vi "InitCCLM.vi"(0 "COM Port Select":refnum<visa-resource-name>, 5 "StartModeEnable":bool=TRUE, 9 "error in (no error)":errorcluster, 11 "User control":T1={"Stimulation Parameters"={"Amplitude (mA)"={"A1"=1, "A2"=0, "A3"=0, "A4"=0, "A5"=0, "A6"=0, "A7"=0, "A8"=0}, "Pulse Width (µs)"={"PW1"=20, "PW2"=20, "PW3"=20, "PW4"=20, "PW5"=20, "PW6"=20, "PW7"=20, "PW8"=20}, "Stimulation Mode"={"M1"=0, "M2"=0, "M3"=0, "M4"=0, "M5"=0, "M6"=0, "M7"=0, "M8"=0}}, "Waveform Parameters"={"Low Frequency Factor"=0, "Main Stim Interval [ms]"=8.0, "Interpulse Interval [ms]"=0, "Channel Execution"=0}, "Active channels"={"C1"=FALSE, "C2"=FALSE, "C3"=FALSE, "C4"=FALSE, "C5"=FALSE, "C6"=FALSE, "C7"=FALSE, "C8"=FALSE}, "LF Active Channels"={"LF1"=FALSE, "LF2"=FALSE, "LF3"=FALSE, "LF4"=FALSE, "LF5"=FALSE, "LF6"=FALSE, "LF7"=FALSE, "LF8"=FALSE}, "Device Control"={"VISA resource name"=""}} {"Stimulation Parameters"."Amplitude (mA)"."A1" max=130; "Stimulation Parameters"."Amplitude (mA)"."A2" max=130; "Stimulation Parameters"."Amplitude (mA)"."A3" max=130; "Stimulation Parameters"."Amplitude (mA)"."A4" max=130; "Stimulation Parameters"."Amplitude (mA)"."A5" max=130; "Stimulation Parameters"."Amplitude (mA)"."A6" max=130; "Stimulation Parameters"."Amplitude (mA)"."A7" max=130; "Stimulation Parameters"."Amplitude (mA)"."A8" max=130; "Stimulation Parameters"."Pulse Width (µs)"."PW1" min=20 max=500; "Stimulation Parameters"."Pulse Width (µs)"."PW2" min=20 max=500; "Stimulation Parameters"."Pulse Width (µs)"."PW3" min=20 max=500; "Stimulation Parameters"."Pulse Width (µs)"."PW4" min=20 max=500; "Stimulation Parameters"."Pulse Width (µs)"."PW5" min=20 max=500; "Stimulation Parameters"."Pulse Width (µs)"."PW6" min=20 max=500; "Stimulation Parameters"."Pulse Width (µs)"."PW7" min=20 max=500; "Stimulation Parameters"."Pulse Width (µs)"."PW8" min=20 max=500; "Stimulation Parameters"."Stimulation Mode"."M8" items=["Singlet", "Doublet", "Triplet"]; "Stimulation Parameters"."Stimulation Mode"."M7" items=["Singlet", "Doublet", "Triplet"]; "Stimulation Parameters"."Stimulation Mode"."M6" items=["Singlet", "Doublet", "Triplet"]; "Stimulation Parameters"."Stimulation Mode"."M5" items=["Singlet", "Doublet", "Triplet"]; "Stimulation Parameters"."Stimulation Mode"."M4" items=["Singlet", "Doublet", "Triplet"]; "Stimulation Parameters"."Stimulation Mode"."M3" items=["Singlet", "Doublet", "Triplet"]; "Stimulation Parameters"."Stimulation Mode"."M2" items=["Singlet", "Doublet", "Triplet"]; "Stimulation Parameters"."Stimulation Mode"."M1" items=["Singlet", "Doublet", "Triplet"]; "Waveform Parameters"."Channel Execution" items=["Fixed Interval", "ASAP"]}) -> (3 "Status":string, 4 "VISA resource name out":refnum<visa-resource-name>, 6 "Stimulation Initialized":bool=TRUE, 14 "CCLM Initialization Error":bool=TRUE, 15 "error out":errorcluster)   [LabVIEW 2020]
uses:
  Type Defs/rs2_ctrl_panel.ctl
panel:
  out "Packet Number Out":i32
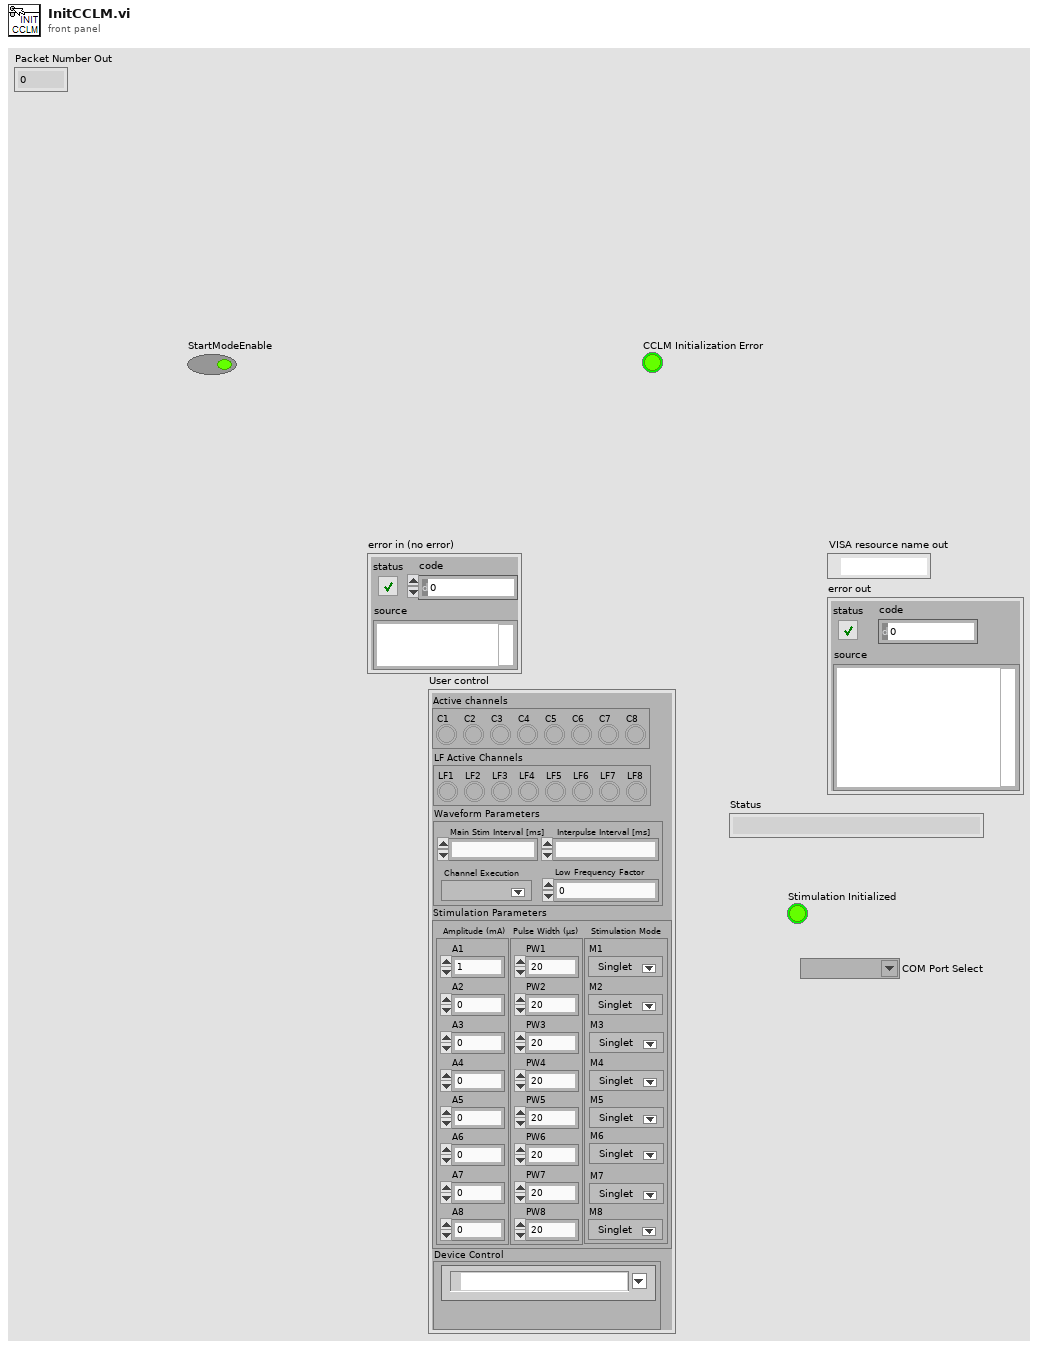
[diagram p1: front panel]
types:
  T1 = typedef "rs2_ctrl_panel.ctl" = cluster{"Stimulation Parameters":cluster{"Amplitude (mA)":cluster{"A1":u8, "A2":u8, "A3":u8, "A4":u8, "A5":u8, "A6":u8, "A7":u8, "A8":u8}, "Pulse Width (µs)":cluster{"PW1":u16, "PW2":u16, "PW3":u16, "PW4":u16, "PW5":u16, "PW6":u16, "PW7":u16, "PW8":u16}, "Stimulation Mode":cluster{"M1":u8, "M2":u8, "M3":u8, "M4":u8, "M5":u8, "M6":u8, "M7":u8, "M8":u8}}, "Waveform Parameters":cluster{"Low Frequency Factor":u8, "Main Stim Interval [ms]":fxp<+,32,11>, "Interpulse Interval [ms]":u8, "Channel Execution":u8}, "Active channels":cluster{"C1":bool, "C2":bool, "C3":bool, "C4":bool, "C5":bool, "C6":bool, "C7":bool, "C8":bool}, "LF Active Channels":cluster{"LF1":bool, "LF2":bool, "LF3":bool, "LF4":bool, "LF5":bool, "LF6":bool, "LF7":bool, "LF8":bool}, "Device Control":cluster{"VISA resource name":refnum<visa-resource-name>}}
  T2 = cluster{"Low Frequency Factor":u8, "Main Stim Interval [ms]":fxp<+,32,11>, "Interpulse Interval [ms]":u8, "Channel Execution":u8}
  T3 = cluster{"C1":bool, "C2":bool, "C3":bool, "C4":bool, "C5":bool, "C6":bool, "C7":bool, "C8":bool}
  T4 = cluster{"LF1":bool, "LF2":bool, "LF3":bool, "LF4":bool, "LF5":bool, "LF6":bool, "LF7":bool, "LF8":bool}
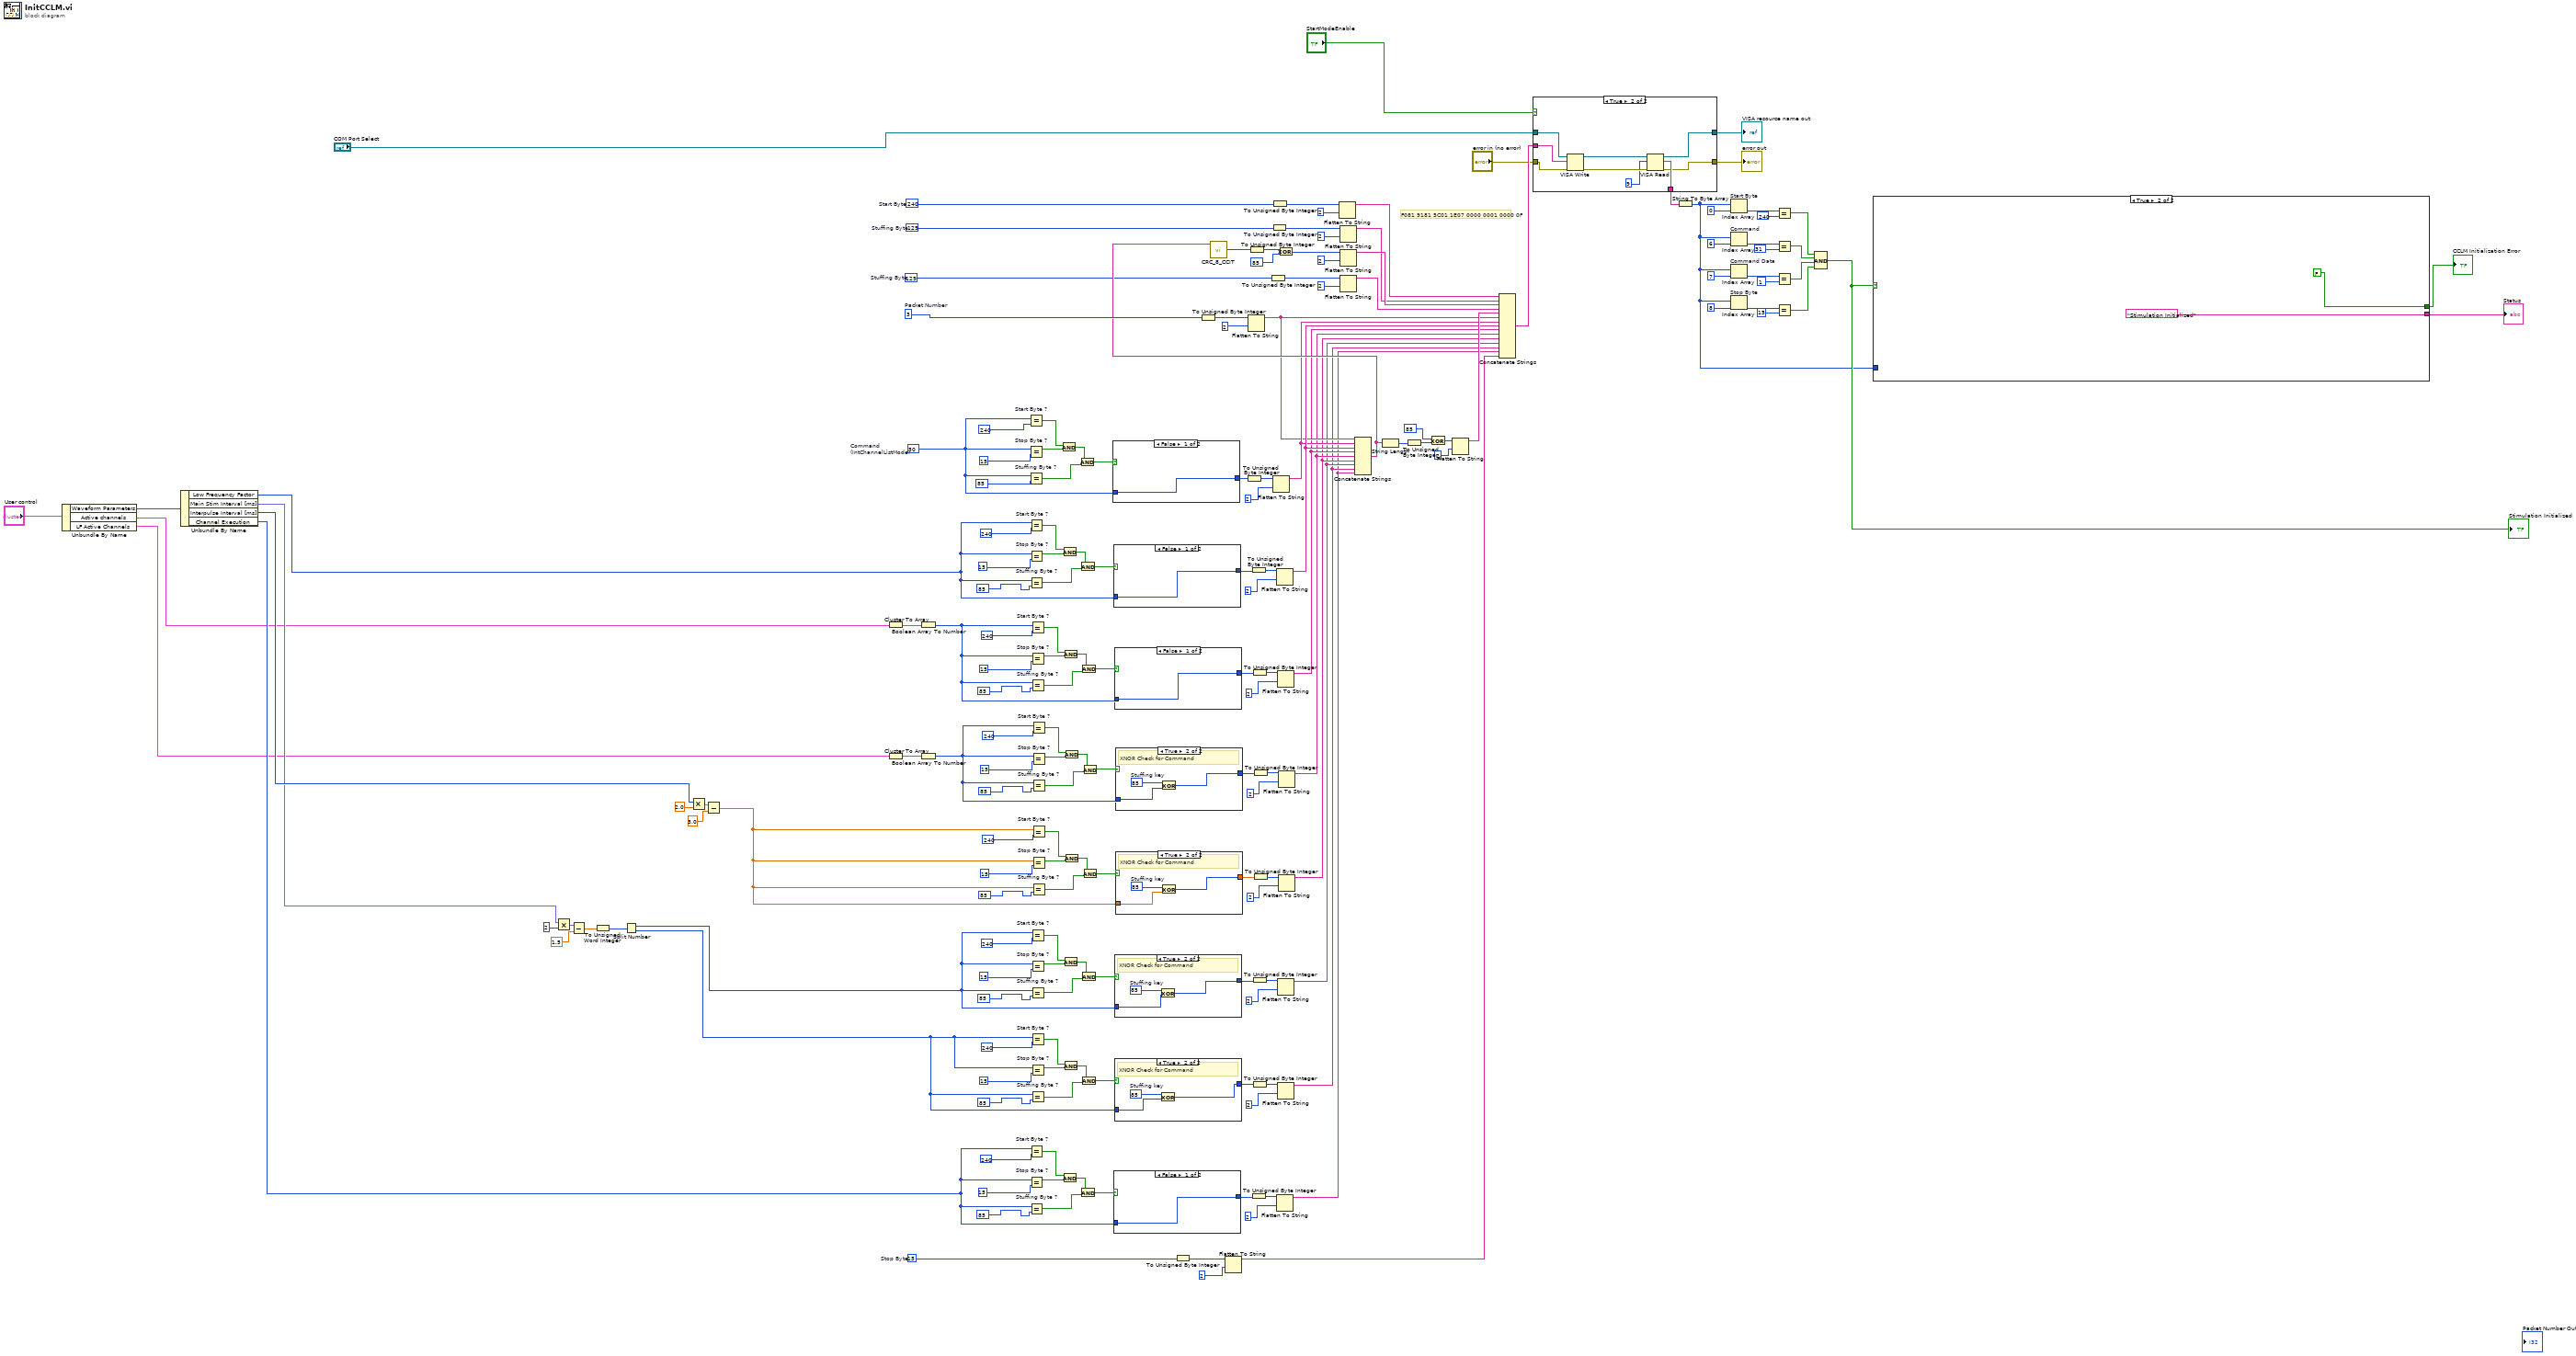
[diagram p0: block diagram]
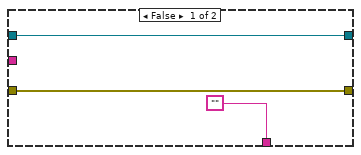
[diagram p2: hidden frame]
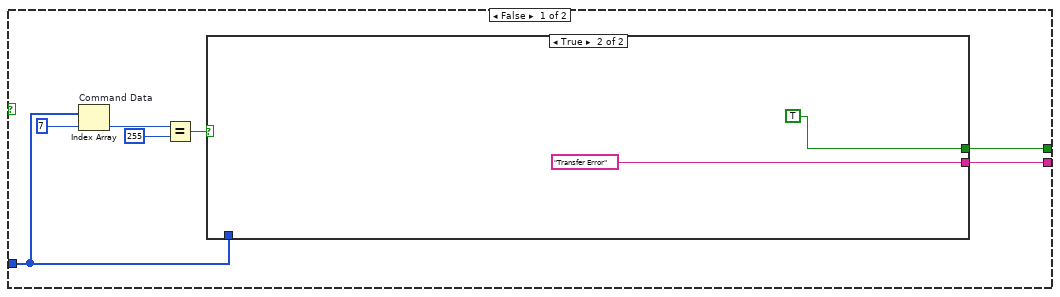
[diagram p3: hidden frame]
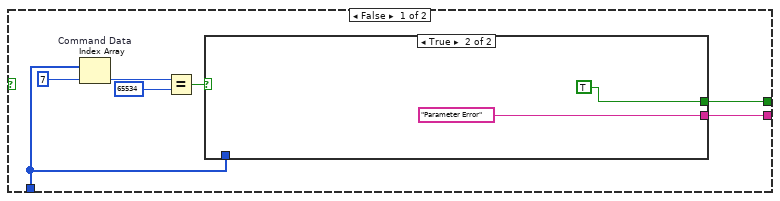
[diagram p4: hidden frame]
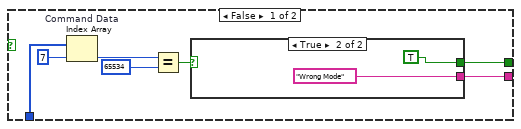
[diagram p5: hidden frame]
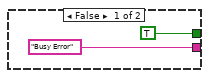
[diagram p6: hidden frame]
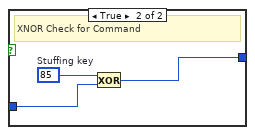
[diagram p7: hidden frame]
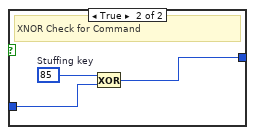
[diagram p12: hidden frame]
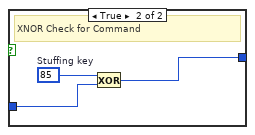
[diagram p13: hidden frame]
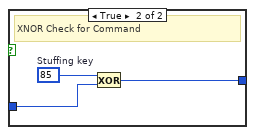
[diagram p14: hidden frame]
diagram:
  w178 = u8 3  # Packet Number
  w135 = 15  # Stop Byte
  w138 = 129  # Stuffing Byte
  w139 = 129  # Stuffing Byte
  w137 = 240  # Start Byte
  w157 = 30  # Command (IntChannelListMode)
  # "F081 9181 5C01 1E07 0000 0001 0000 0F"
  n1 = Unbundle By Name("User control") -> ("Waveform Parameters"=w10:T2, "Active channels"=w5:T3, "LF Active Channels"=w4:T4)
  n2 = Unbundle By Name(w10) -> ("Low Frequency Factor"=w9:u8, "Main Stim Interval [ms]"=w7:fxp<+,32,11>, "Interpulse Interval [ms]"=w8:u8, "Channel Execution"=w6:u8)
  n3 = Multiply(x=w7, y=u8 2) -> (x*y=w35:fxp<+,40,19>)
  n4 = Subtract(x=w35, y=1.5) -> (x-y=w32:dbl)
  n5 = To Unsigned Word Integer(number=w32) -> (unsigned 16bit integer=w33:u16)
  n6 = Split Number(x=w33) -> (hi(x)=w39:u8, lo(x)=w38:u8)
  n7 = Multiply(x=w8, y=2.0) -> (x*y=w42:dbl)
  n8 = Subtract(x=w42, y=3.0) -> (x-y=w40:dbl)
  n9 = Cluster To Array(cluster=w5) -> (array=w48:bool[])
  n10 = Cluster To Array(cluster=w4) -> (array=w44:bool[])
  n11 = Boolean Array To Number(Boolean array=w48) -> (number=w46:u8)
  n12 = Boolean Array To Number(Boolean array=w44) -> (number=w47:u8)
  n13 = Equal? "Start Byte ?"(x=w157, y=240 ("IntAck")) -> (x = y?=w121:bool)
  n14 = Equal? "Stop Byte ?"(x=w157, y=15 ("IntAck")) -> (x = y?=w122:bool)
  n15 = Equal? "Stuffing Byte ?"(x=w157, y=85 ("IntAck")) -> (x = y?=w124:bool)
  n16 = Equal? "Start Byte ?"(x=w9, y=240 ("IntAck")) -> (x = y?=w126:bool)
  n17 = Equal? "Stop Byte ?"(x=w9, y=15 ("IntAck")) -> (x = y?=w127:bool)
  n18 = Equal? "Stuffing Byte ?"(x=w9, y=85 ("IntAck")) -> (x = y?=w129:bool)
  n19 = Equal? "Start Byte ?"(x=w6, y=240 ("IntAck")) -> (x = y?=w56:bool)
  n20 = Equal? "Stop Byte ?"(x=w6, y=15 ("IntAck")) -> (x = y?=w57:bool)
  n21 = Equal? "Stuffing Byte ?"(x=w6, y=85 ("IntAck")) -> (x = y?=w59:bool)
  n22 = Equal? "Start Byte ?"(x=w46, y=240 ("IntAck")) -> (x = y?=w110:bool)
  n23 = Equal? "Stop Byte ?"(x=w46, y=15 ("IntAck")) -> (x = y?=w111:bool)
  n24 = Equal? "Stuffing Byte ?"(x=w46, y=85 ("IntAck")) -> (x = y?=w113:bool)
  n25 = Equal? "Start Byte ?"(x=w39, y=240 ("IntAck")) -> (x = y?=w77:bool)
  n26 = Equal? "Stop Byte ?"(x=w39, y=15 ("IntAck")) -> (x = y?=w78:bool)
  n27 = Equal? "Stuffing Byte ?"(x=w39, y=85 ("IntAck")) -> (x = y?=w80:bool)
  n28 = Equal? "Start Byte ?"(x=w38, y=240 ("IntAck")) -> (x = y?=w67:bool)
  n29 = Equal? "Stop Byte ?"(x=w38, y=15 ("IntAck")) -> (x = y?=w68:bool)
  n30 = Equal? "Stuffing Byte ?"(x=w38, y=85 ("IntAck")) -> (x = y?=w70:bool)
  n31 = Equal? "Start Byte ?"(x=w47, y=240 ("IntAck")) -> (x = y?=w99:bool)
  n32 = Equal? "Stop Byte ?"(x=w47, y=15 ("IntAck")) -> (x = y?=w100:bool)
  n33 = Equal? "Stuffing Byte ?"(x=w47, y=85 ("IntAck")) -> (x = y?=w102:bool)
  n34 = Equal? "Start Byte ?"(x=w40, y=240 ("IntAck")) -> (x = y?=w88:bool)
  n35 = Equal? "Stop Byte ?"(x=w40, y=15 ("IntAck")) -> (x = y?=w89:bool)
  n36 = Equal? "Stuffing Byte ?"(x=w40, y=85 ("IntAck")) -> (x = y?=w91:bool)
  n37 = And(x=w121, y=w122) -> (x .and. y?=w123:bool)
  n38 = And(x=w126, y=w127) -> (x .and. y?=w128:bool)
  n39 = And(x=w56, y=w57) -> (x .and. y?=w58:bool)
  n40 = And(x=w110, y=w111) -> (x .and. y?=w112:bool)
  n41 = And(x=w77, y=w78) -> (x .and. y?=w79:bool)
  n42 = And(x=w67, y=w68) -> (x .and. y?=w69:bool)
  n43 = And(x=w99, y=w100) -> (x .and. y?=w101:bool)
  n44 = And(x=w88, y=w89) -> (x .and. y?=w90:bool)
  n45 = And(x=w123, y=w124) -> (x .and. y?=w125:bool)
  n46 = And(x=w128, y=w129) -> (x .and. y?=w130:bool)
  n47 = And(x=w58, y=w59) -> (x .and. y?=w60:bool)
  n48 = And(x=w112, y=w113) -> (x .and. y?=w114:bool)
  n49 = And(x=w79, y=w80) -> (x .and. y?=w81:bool)
  n50 = And(x=w69, y=w70) -> (x .and. y?=w71:bool)
  n51 = And(x=w101, y=w102) -> (x .and. y?=w103:bool)
  n52 = And(x=w90, y=w91) -> (x .and. y?=w92:bool)
  n53 = case shown="False" w125 {
    tunnel: w157 -> [w181 w184]
    tunnel: [w181 w182] -> w159
    frame False {
    }
    frame True {
      w183 = 85  # Stuffing key
      # "XNOR Check for Command"
      n54 = Exclusive Or(1:w184, 2:w183) -> (0:w182:i32)
    }
  }
  n55 = case shown="False" w130 {
    tunnel: w9 -> [w185 w188]
    tunnel: [w185 w186] -> w158
    frame False {
    }
    frame True {
      w187 = 85  # Stuffing key
      # "XNOR Check for Command"
      n56 = Exclusive Or(1:w188, 2:w187) -> (0:w186:i32)
    }
  }
  n57 = case shown="False" w60 {
    tunnel: w6 -> [w189 w192]
    tunnel: [w189 w190] -> w65
    frame False {
    }
    frame True {
      w191 = 85  # Stuffing key
      # "XNOR Check for Command"
      n58 = Exclusive Or(1:w192, 2:w191) -> (0:w190:i32)
    }
  }
  n59 = case shown="False" w114 {
    tunnel: w46 -> [w193 w196]
    tunnel: [w193 w194] -> w119
    frame False {
    }
    frame True {
      w195 = 85  # Stuffing key
      # "XNOR Check for Command"
      n60 = Exclusive Or(1:w196, 2:w195) -> (0:w194:i32)
    }
  }
  n61 = case shown="True" w81 {
    tunnel: w39 -> [w197 w198]
    tunnel: [w197 w199] -> w86
    frame False {
    }
    frame True {
      w200 = 85  # Stuffing key
      # "XNOR Check for Command"
      n62 = Exclusive Or(1:w198, 2:w200) -> (0:w199:i32)
    }
  }
  n63 = case shown="True" w71 {
    tunnel: w38 -> [w201 w203]
    tunnel: [w201 w202] -> w37
    frame False {
    }
    frame True {
      w204 = 85  # Stuffing key
      # "XNOR Check for Command"
      n64 = Exclusive Or(1:w203, 2:w204) -> (0:w202:i32)
    }
  }
  n65 = case shown="True" w103 {
    tunnel: w47 -> [w205 w208]
    tunnel: [w205 w206] -> w108
    frame False {
    }
    frame True {
      w207 = 85  # Stuffing key
      # "XNOR Check for Command"
      n66 = Exclusive Or(1:w208, 2:w207) -> (0:w206:i32)
    }
  }
  n67 = case shown="True" w92 {
    tunnel: w40 -> [w209 w212]
    tunnel: [w209 w210] -> w97
    frame False {
    }
    frame True {
      w211 = 85  # Stuffing key
      # "XNOR Check for Command"
      n68 = Exclusive Or(1:w212, 2:w211) -> (0:w210:i32)
    }
  }
  n69 = To Unsigned Byte Integer(number=w135) -> (unsigned 8bit integer=w136:u8)
  n70 = To Unsigned Byte Integer(number=w178) -> (unsigned 8bit integer=w168:u8)
  n71 = Flatten To String(anything=w136, byte order (0:big-endian, network order)=2) -> (data string=w49:string)  [unwired: 2 in, 2 out]
  n72 = To Unsigned Byte Integer(number=w159) -> (unsigned 8bit integer=w167:u8)
  n73 = Flatten To String(anything=w168, byte order (0:big-endian, network order)=2) -> (data string=w160:string)  [unwired: 2 in, 2 out]
  n74 = To Unsigned Byte Integer(number=w158) -> (unsigned 8bit integer=w166:u8)
  n75 = To Unsigned Byte Integer(number=w65) -> (unsigned 8bit integer=w66:u8)
  n76 = To Unsigned Byte Integer(number=w119) -> (unsigned 8bit integer=w120:u8)
  n77 = To Unsigned Byte Integer(number=w86) -> (unsigned 8bit integer=w87:u8)
  n78 = To Unsigned Byte Integer(number=w37) -> (unsigned 8bit integer=w76:u8)
  n79 = To Unsigned Byte Integer(number=w108) -> (unsigned 8bit integer=w109:u8)
  n80 = To Unsigned Byte Integer(number=w97) -> (unsigned 8bit integer=w98:u8)
  n81 = To Unsigned Byte Integer(number=w139) -> (unsigned 8bit integer=w142:u8)
  n82 = To Unsigned Byte Integer(number=w138) -> (unsigned 8bit integer=w141:u8)
  n83 = To Unsigned Byte Integer(number=w137) -> (unsigned 8bit integer=w140:u8)
  n84 = Flatten To String(anything=w167, byte order (0:big-endian, network order)=2) -> (data string=w161:string)  [unwired: 2 in, 2 out]
  n85 = Flatten To String(anything=w166, byte order (0:big-endian, network order)=2) -> (data string=w162:string)  [unwired: 2 in, 2 out]
  n86 = Flatten To String(anything=w66, byte order (0:big-endian, network order)=2) -> (data string=w50:string)  [unwired: 2 in, 2 out]
  n87 = Flatten To String(anything=w120, byte order (0:big-endian, network order)=2) -> (data string=w55:string)  [unwired: 2 in, 2 out]
  n88 = Flatten To String(anything=w87, byte order (0:big-endian, network order)=2) -> (data string=w52:string)  [unwired: 2 in, 2 out]
  n89 = Flatten To String(anything=w76, byte order (0:big-endian, network order)=2) -> (data string=w51:string)  [unwired: 2 in, 2 out]
  n90 = Flatten To String(anything=w109, byte order (0:big-endian, network order)=2) -> (data string=w54:string)  [unwired: 2 in, 2 out]
  n91 = Flatten To String(anything=w98, byte order (0:big-endian, network order)=2) -> (data string=w53:string)  [unwired: 2 in, 2 out]
  n92 = Flatten To String(anything=w140, byte order (0:big-endian, network order)=2) -> (data string=w131:string)  [unwired: 2 in, 2 out]
  n93 = Flatten To String(anything=w141, byte order (0:big-endian, network order)=2) -> (data string=w132:string)  [unwired: 2 in, 2 out]
  n94 = Flatten To String(anything=w142, byte order (0:big-endian, network order)=2) -> (data string=w134:string)  [unwired: 2 in, 2 out]
  n95 = Concatenate Strings(w160, w161, w162, w55, w54, w53, w52, w51, w50) -> (w170:string)
  n96 = call "CRC_8_CCIT.vi"("Data String"=w170) -> ("Numeric"=w169:u8)  [unwired: 10 in]
  n97 = To Unsigned Byte Integer(number=w169) -> (unsigned 8bit integer=w172:u8)
  n98 = Exclusive Or(1:u8 85, 2:w172) -> (0:w171:u8)
  n99 = Flatten To String(anything=w171, byte order (0:big-endian, network order)=2) -> (data string=w133:string)  [unwired: 2 in, 2 out]
  n100 = String Length(string=w170) -> (length=w164:i32)
  n101 = To Unsigned Byte Integer(number=w164) -> (unsigned 8bit integer=w175:u8)
  n102 = Exclusive Or(1:w175, 2:u8 85) -> (0:w174:u8)
  n103 = Flatten To String(anything=w174, byte order (0:big-endian, network order)=2) -> (data string=w165:string)  [unwired: 2 in, 2 out]
  n104 = Concatenate Strings(w131, w132, w133, w134, w165, w160, w161, w162, w55, w54, w53, w52, w51, w50, w49) -> (w45:string)
  n105 = case shown="True" "StartModeEnable" {
    tunnel: "COM Port Select" -> [w213 w224]
    tunnel: w45 -> [_ w223]
    tunnel: ["" w222] -> w15
    tunnel: "error in (no error)" -> [w214 w218]
    tunnel: [w213 w217] -> w12
    tunnel: [w214 w216] -> w11
    frame False {
    }
    frame True {
      n106 = VISA Write(VISA resource name=w224, write buffer=w223, error in (no error)=w218) -> (VISA resource name out=w221:refnum<visa-resource-name>, error out=w220:errorcluster)  [unwired: 1 out]
      n107 = VISA Read(VISA resource name=w221, byte count=u32 9, error in (no error)=w220) -> (VISA resource name out=w217:refnum<visa-resource-name>, read buffer=w222:string, error out=w216:errorcluster)  [unwired: 1 out]
    }
  }
  "VISA resource name out" <- w12
  "error out" <- w11
  n108 = String To Byte Array(string=w15) -> (unsigned byte array=w14:u8[])
  n109 = Index Array "Start Byte"(array=w14, index=0) -> (element=w26:u8)
  n110 = Index Array "Command"(array=w14, index=6) -> (element=w22:u8)
  n111 = Index Array "Command Data"(array=w14, index=7) -> (element=w21:u8)
  n112 = Index Array "Stop Byte"(array=w14, index=8) -> (element=w20:u8)
  n113 = Equal?(x=w26, y=u16 240) -> (x = y?=w19:bool)
  n114 = Equal?(x=w22, y=u16 31) -> (x = y?=w18:bool)
  n115 = Equal?(x=w21, y=u16 1) -> (x = y?=w17:bool)
  n116 = Equal?(x=w20, y=u16 15) -> (x = y?=w16:bool)
  n117 = Compound Arithmetic op=AND(w19, w18, w17, w16) -> (w179:bool)
  "Stimulation Initialized" <- w179
  n118 = case shown="True" w179 {
    tunnel: [w227 "Stimulation Initialized"] -> w180
    tunnel: w14 -> [w226 _]
    tunnel: [w225 FALSE] -> w1
    frame False {
      n119 = Index Array "Command Data"(array=w226, index=7) -> (element=w229:u8)
      n120 = Equal?(x=w229, y=u16 255) -> (x = y?=w228:bool)
      n121 = case shown="True" w228 {
        tunnel: [w234 "Transfer Error"] -> w227
        tunnel: w226 -> [w233 _]
        tunnel: [w232 TRUE] -> w225
        frame False {
          n122 = Index Array "Command Data"(array=w233, index=7) -> (element=w236:u8)
          n123 = Equal?(x=w236, y=u16 65534) -> (x = y?=w235:bool)
          n124 = case shown="True" w235 {
            tunnel: [w240 "Parameter Error"] -> w234
            tunnel: w233 -> [w242 _]
            tunnel: [w239 TRUE] -> w232
            frame False {
              n125 = Index Array "Command Data"(array=w242, index=7) -> (element=w243:u8)
              n126 = Equal?(x=w243, y=u16 65534) -> (x = y?=w241:bool)
              n127 = case shown="True" w241 {
                tunnel: ["Busy Error" "Wrong Mode"] -> w240
                tunnel: [TRUE TRUE] -> w239
                frame False {
                }
                frame True {
                }
              }
            }
            frame True {
            }
          }
        }
        frame True {
        }
      }
    }
    frame True {
    }
  }
  "Status" <- w180
  "CCLM Initialization Error" <- w1
